vi "Connection Engine.vi"(8 "error in (no error)":errorcluster, 11 "State Variables":T1) -> (0 "error out":errorcluster)   [LabVIEW 2013, in "Control Addon Engine.lvlib" / "Network Common API.lvlib"]
uses:
  Network Common API.lvlib
  Inline Async API/Controls/Engine State Variables.ctl
  TCP Refs.ctl
  Network Comm Global Ref.ctl
  Stop FG/Stop Global Ref.ctl
  Stop FG/Stop Global Commands.ctl
  <userlib>/STM/TCP/stm_TCP Read Options.ctl
  <userlib>/STM/Connection Manager/TCP/stm_TCPConnectionMethod.ctl
  <userlib>/STM/Connection Manager/TCP/stm_TCPConnectionProperties.ctl
  <userlib>/STM/TCP/STM Read Meta Data (TCP Ref).vi
  <userlib>/STM/TCP/STM Get Connection Reference (TCP).vi
  <vilib>/NI Veristand/Custom Device Tools/Custom Device Utility Library/Custom Device Utility Library.lvlib
  Stop FG/Stop FG.lvlib
  Inline Async API/Inline Async API.lvlib
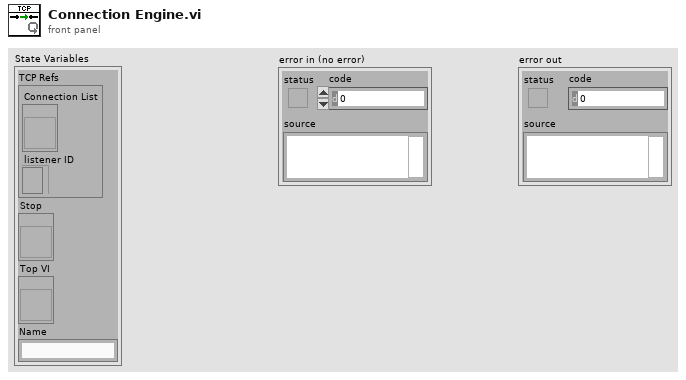
[diagram p1: front panel]
types:
  T1 = typedef "Control Addon Engine.lvlib/Inline Async API.lvlib/Engine State Variables.ctl" = cluster{"TCP Refs":T2, "Stop":T4, "Top VI":refnum<vi>, "Name":string}
  T2 = typedef "Control Addon Engine.lvlib/Network Common API.lvlib/TCP Refs.ctl" = cluster{"Connection List":T3, "listener ID":refnum<k5>}
  T3 = typedef "Control Addon Engine.lvlib/Network Common API.lvlib/Network Comm Global Ref.ctl" = refnum<vi>
  T4 = typedef "Control Addon Engine.lvlib/Stop FG.lvlib/Stop Global Ref.ctl" = refnum<vi>
  T5 = typedef "Control Addon Engine.lvlib/Stop FG.lvlib/Stop Global Commands.ctl" = enum16{"Write", "Read", "Reset"}
  T6 = typedef "stm_TCP Read Options.ctl" = cluster{"Ignore Timeout Error":bool, "timeout ms (1000)":i32}
  T7 = typedef "stm_TCPConnectionProperties.ctl" = cluster{"Name":string, "Address":string, "Custom":string}
  T8 = typedef "stm_TCPConnectionMethod.ctl" = enum16{"Initialize", "Add Connection", "Set Properties", "Get Connection(s)", "Remove Connection", "Remove All Connections", "Get Connection Count"}
  T9 = typedef "stm_TCP Connection Info.ctl" = cluster{"connection ID":refnum<k5>, "Meta data":T10[]}
  T10 = typedef "stm_MetaDataElement.ctl" = string
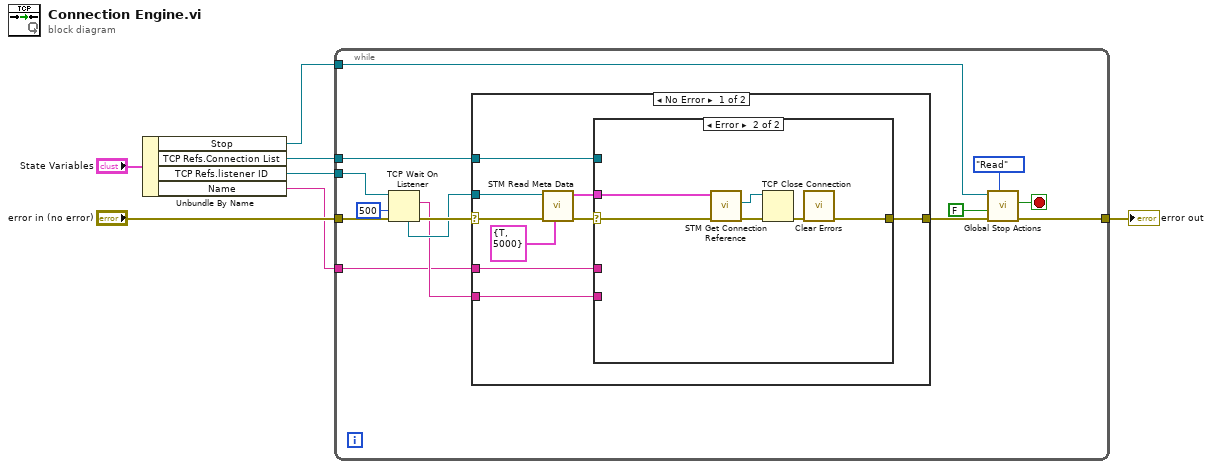
[diagram p0: block diagram]
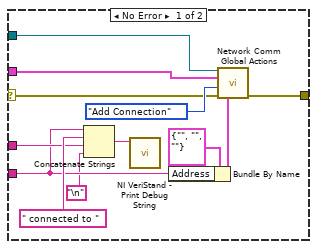
[diagram p2: hidden frame]
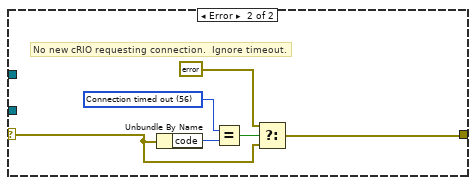
[diagram p3: hidden frame]
diagram:
  n1 = Unbundle By Name("State Variables") -> ("Stop"=w7:T4, "TCP Refs.Connection List"=w5:T3, "TCP Refs.listener ID"=w6:refnum<k5>, "Name"=w1:string)
  n2 = while {
    tunnel: "error in (no error)" -> [w21]
    tunnel: w6 -> [w20]
    tunnel: w7 -> [w13]
    tunnel: [w8] -> w2
    tunnel: w5 -> [w11]
    tunnel: w1 -> [w10]
    stop <- w15 stop-if-true
    n3 = TCP Wait On Listener(8:w21, 9:500 ("timeout ms (wait forever: -1)"), 11:w20) -> (0:w18:errorcluster, 2:w16:string, 4:w17:refnum<k5>)  [unwired: 1 in, 2 out]
    n4 = case shown="No Error" w18 {
      selector: w18 -> [w30 w50]
      tunnel: w17 -> [w25 _]
      tunnel: [w29 w51] -> w14
      tunnel: w16 -> [w27 _]
      tunnel: w11 -> [w28 _]
      tunnel: w10 -> [w26 _]
      frame No Error {
        n5 = call-poly <userlib>:"STM Read Meta Data.vi"("Options"=T6 {"Ignore Timeout Error"=TRUE, "timeout ms (1000)"=5000} ("options"), "error in"=w30, "connection ID"=w25) -> ("error out"=w24:errorcluster, "Connection Info Out"=w23:T9)  [unwired: 6 in, 1 out]
        n6 = case shown="Error" w24 {
          selector: w24 -> [w38 w45]
          tunnel: w28 -> [w36 _]
          tunnel: w23 -> [w37 w46]
          tunnel: [w39 w48] -> w29
          tunnel: w27 -> [w32 _]
          tunnel: w26 -> [w33 _]
          frame No Error {
            n7 = Concatenate Strings(w32, " connected to " ("string"), w33, "\n") -> (w34:string)
            n8 = call <vilib>:"NI VeriStand - Print Debug String.vi"("Message"=w34) -> ()  [unwired: 10 in, 1 out]
            n9 = Bundle By Name(cluster=T7 {"Name"="", "Address"="", "Custom"=""} ("Properties In"), "Address"=w32) -> (w42:T7)
            n10 = call "Network Comm Global Actions.vi"("ref in"=w36, "Connection In"=w37, "Method"=stm_TCPConnectionMethod."Add Connection", "error in (no error)"=w38, "Properties In"=w42) -> ("error out"=w39:errorcluster)  [unwired: 4 in, 6 out]
          }
          frame Error {
            n11 = call-poly <userlib>:"STM Get Connection Reference.vi"("error in"=w45, "Connection Info"=w46) -> ("error out"=w43:errorcluster, "connection ID out"=w44:refnum<k5>)  [unwired: 7 in, 1 out]
            n12 = TCP Close Connection(connection ID=w44, error in (no error)=w43) -> (error out=w47:errorcluster)  [unwired: 1 in, 1 out]
            n13 = call <vilib>:"Clear Errors.vi"("error in (no error)"=w47) -> ("error out"=w48:errorcluster)  [unwired: 6 in]
          }
        }
      }
      frame Error {
        w49 = 56 items=["No Error", "Argument Error", "Memory Full", "Out of Zone", "End of File", "File Already Open", "Generic File IO Error", "File Not Found", "File Permission Error", "Disk Full", "Duplicate Path", "Too Many Files Open", "Not Enabled", "Resource File Not Found", "Cannot Add Resource", "Resource Not Found", "Image Not Found", "Image Memory Error", "Pen Does Not Exist", "Config Bad Type", "Config Token Not Found", "Config Parse Error", "Config Memory Error", "Bad External Code Format", "Bad External Code Offset", "External Code Not Present", "Null Window", "Destroy Window Mixup", "Null Menu", "Print Aborted", "Bad Print Record", "Print Driver Error", "Windows Error During Print", "Memory Error During Print", "Print Dialog Error", "Generic Print Error", "Invalid Device Refnum", "Device Not Found", "Device Parameter Error", "Device Unit Error", "Can't Open Device", "Device Call Aborted", "Generic Error", "Cancelled By User", "Object ID Too Low", "Object ID Too High", "Object Not In Heap", "Unknown Heap", "Bad DefProc ID", "DefProc Not In Table", "Message Out Of Range", "Null Method", "Unknown Message", "Manager Call Not Supported", "Bad address", "Connection In progress", "Connection timed out", "Connection is already in progress", "Network attribute not supported", "Network error", "Address in use", "System out of memory", "Connection aborted", "Connection refused", "Connection is not connected", "Connection is already connected", "Connection closed", "Initialize error (interapplication manager)", "Bad occurrence", "Wait on unbound occurrence handler", "Occurrence queue overflow", "Bad path", "Semaphore not signaled", "Unrecognized type (interapplication manager)"] ("1st Error to Convert")
        # "No new cRIO requesting connection.  Ignore timeout."
        n14 = Unbundle By Name(w50) -> ("code"=w53:i32)
        n15 = Equal?(x=w49, y=w53) -> (x = y?=w54:bool)
        n16 = Select(t=errorcluster {"status"=FALSE, "code"=0, "source"=""} ("error in (no error)"), s=w54, f=w50) -> (s? t:f=w51:errorcluster)
      }
    }
    n17 = call "Global Stop Actions.vi"("Command"=Stop_Global_Commands."Read", "error in (no error)"=w14, "Stop on Error?"=FALSE, "vi reference"=w13) -> ("error out"=w8:errorcluster, "Latched Stop"=w15:bool)  [unwired: 5 in, 1 out]
  }
  "error out" <- w2
